vi "SSL Log Reader.vi"(9 "Slide":i64(slide) min=0 max=778291377 scale=0.0..778291377.0, 10 "Boolean 4":bool, 11 "file path (use dialog)":path=path "E:/Media/2016-07-01_cmdragons_immortals.log") -> (0 "error out":errorcluster, 1 "Playing":bool, 2 "channel 2":T1, 3 "Channel out":T1, 4 "size (in bytes)":i64, 6 "offset (in bytes)":i64)   [LabVIEW 2016]
uses:
  <extravilib>/ChannelInstances/Stream-a[.](u8)/)Channel.ctl
  <extravilib>/ChannelInstances/Stream-a[.](u8)/Write With Abort.vi
  <extravilib>/ChannelInstances/Stream-a[.](u8)/Endpoint.vi
  <extravilib>/ChannelInstances/Stream-a[.](u8)/)Channel.vi
  <resource>/ChannelSupport/_ChannelSupport/WaitIfNeeded.vi
  <extravilib>/ChannelInstances/Stream-a[.](u8).lvlib
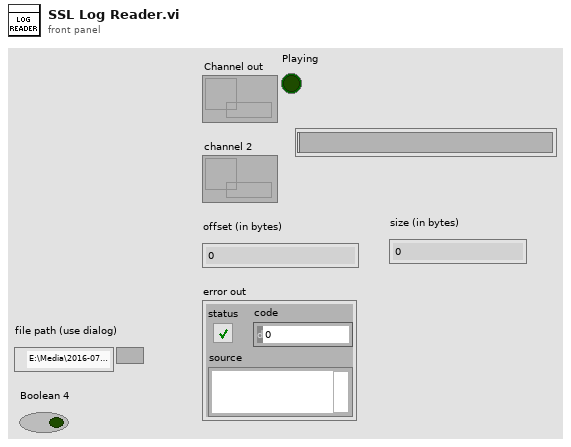
[diagram p1: front panel]
types:
  T1 = typedef "Stream-a[.](u8).lvlib/)Channel.ctl" = refnum<queue>
  T2 = enum16{"open", "replace", "create", "open or create", "replace or create", "replace or create with confirmation"}
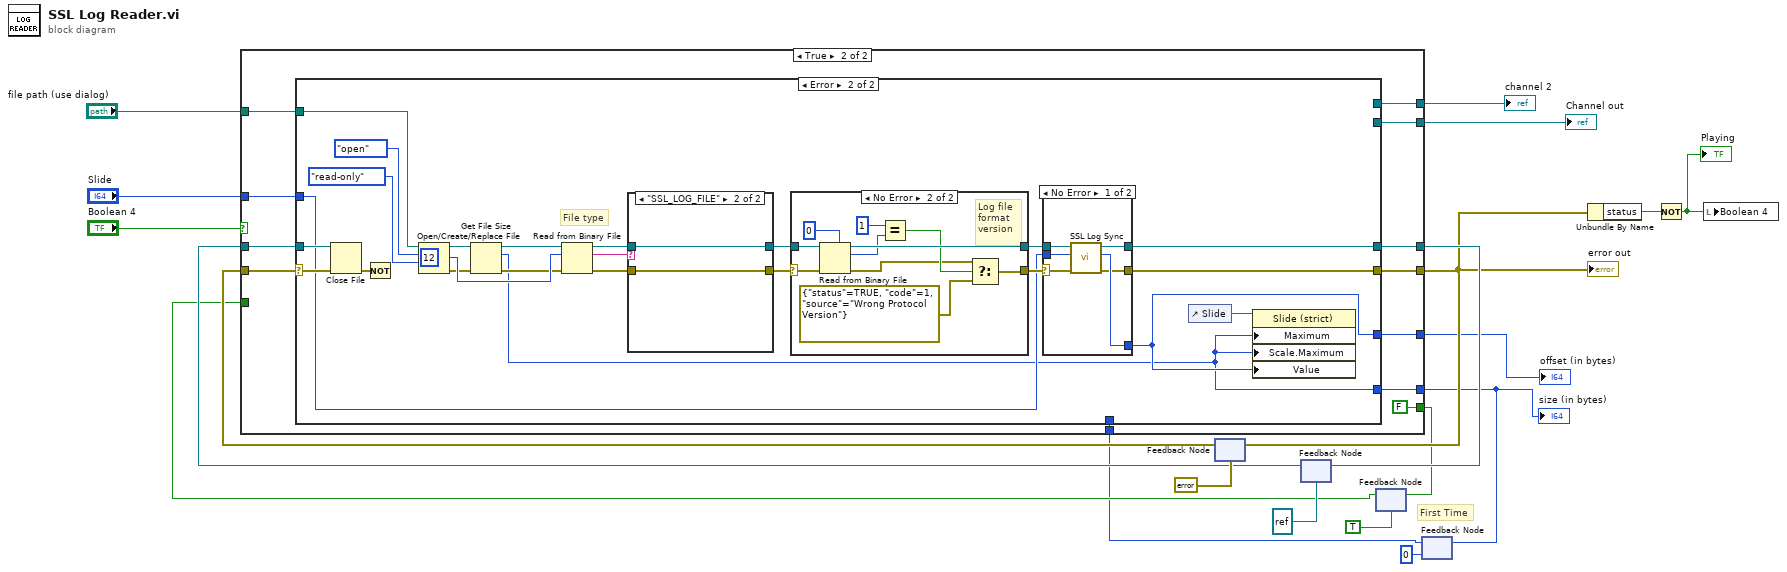
[diagram p0: block diagram]
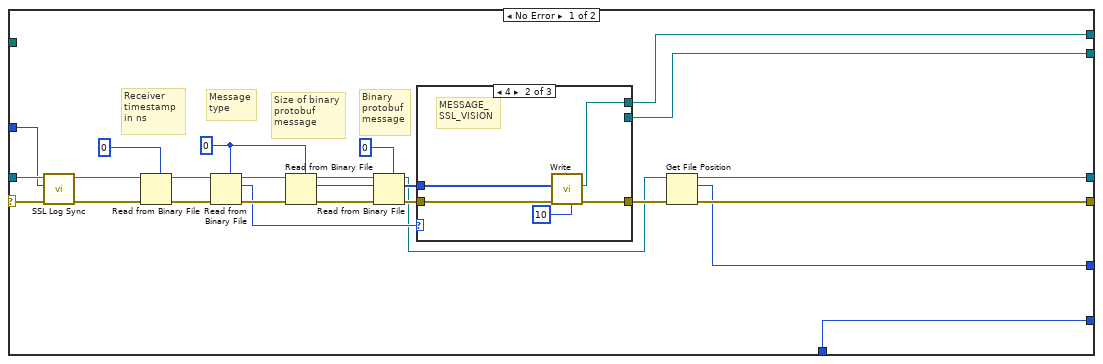
[diagram p3: hidden frame]
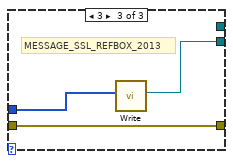
[diagram p5: hidden frame]
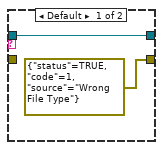
[diagram p7: hidden frame]
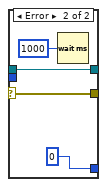
[diagram p8: hidden frame]
diagram:
  # "First Time"
  n1 = feedback #1(errorcluster {"status"=FALSE, "code"=0, "source"=""} ("error out")) -> (w13:errorcluster)
  n2 = feedback #2(refnum<file> refnum ("refnum out")) -> (w11:refnum<file>)
  n3 = feedback #3(TRUE) -> (w6:bool)
  n4 = feedback #4(i64 0 ("size (in bytes)")) -> (w1:i64)
  n5 = case shown="True" "Boolean 4" {
    tunnel: [w23 w37] -> w4
    tunnel: "file path (use dialog)" -> [_ w36]
    tunnel: [_ w35] -> w19
    tunnel: [_ w34] -> w18
    tunnel: "Slide" -> [w23 w31]
    tunnel: [w24 w33] -> w9
    tunnel: w13 -> [w24 w29]
    tunnel: [w25 w32] -> w12
    tunnel: w11 -> [w25 w30]
    tunnel: [w22 FALSE] -> w7
    tunnel: w6 -> [w22 _]
    tunnel: [w21 w27] -> w3
    tunnel: w1 -> [w21 w26]
    frame False {
    }
    frame True {
      n6 = case shown="Error" w29 {
        selector: w29 -> [w48 w78]
        tunnel: [w44 w81] -> w33
        tunnel: [w63 _] -> w34
        tunnel: [w62 _] -> w35
        tunnel: w36 -> [_ w88]
        tunnel: [w39 w74] -> w37
        tunnel: [w42 w79] -> w32
        tunnel: w30 -> [w47 w77]
        tunnel: w31 -> [w46 w75]
        tunnel: [w38 w72] -> w27
        tunnel: w26 -> [w38 _]
        frame No Error {
          w53 = 0 ("data type")
          # "Binary\nprotobuf\nmessage"
          # "Size of binary\nprotobuf \nmessage"
          # "Receiver \ntimestamp \nin ns"
          # "Message\ntype"
          n7 = call "SSL Log Sync.vi"("error in (no error)"=w48, "Slide"=w46, "Byte Stream File in"=w47) -> ("error out"=w40:errorcluster, "Byte Stream File out"=w41:refnum<file>)  [unwired: 6 in, 1 out]
          n8 = Read from Binary File(5:i64 0 ("data type"), 8:w40, 11:w41) -> (0:w58:errorcluster, 3:w59:refnum<file>)  [unwired: 3 in, 2 out]
          n9 = Read from Binary File(5:w53, 8:w58, 11:w59) -> (0:w55:errorcluster, 2:w49:i32, 3:w57:refnum<file>)  [unwired: 3 in, 1 out]
          n10 = Read from Binary File(5:w53, 8:w55, 11:w57) -> (0:w54:errorcluster, 2:w50:i32, 3:w56:refnum<file>)  [unwired: 3 in, 1 out]
          n11 = Read from Binary File(5:u8 0 ("data type"), 8:w54, 10:w50, 11:w56) -> (0:w51:errorcluster, 2:w52:u8[], 3:w43:refnum<file>)  [unwired: 2 in, 1 out]
          n12 = case shown="4" w49 {
            tunnel: w52 -> [_ w68 w70]
            tunnel: w51 -> [w64 w67 w71]
            tunnel: [w64 w67 w71] -> w45
            tunnel: [_ w66 _] -> w63
            tunnel: [_ _ w69] -> w62
            frame Default {
            }
            frame 4 {
              # "MESSAGE_\nSSL_VISION"
              n13 = call <extravilib>:"Write.vi"("size (unlimited)"=10, "element"=w68) -> ("channel"=w66:T1)  [unwired: 7 in, 2 out]
            }
            frame 3 {
              # "MESSAGE_SSL_REFBOX_2013"
              n14 = call <extravilib>:"Write.vi"("element"=w70) -> ("channel"=w69:T1)  [unwired: 8 in, 2 out]
            }
          }
          n15 = Get File Position(4:w45, 7:w43) -> (0:w44:errorcluster, 2:w39:i64, 3:w42:refnum<file>)
        }
        frame Error {
          # "File type"
          n16 = Close File(refnum=w77, error in=w78) -> (error out=w76:errorcluster)  [unwired: 1 out]
          n17 = Not(x=w76) -> ()  [unwired: 1 out]
          n18 = Open/Create/Replace File(file path (use dialog)=w88, operation (0:open)=T2."open", access (0:read/write)=enum16{"read/write", "read-only", "write-only"}."read-only") -> (refnum out=w92:refnum<file>, error out=w89:errorcluster)  [unwired: 3 in, 1 out]
          n19 = Get File Size(file=w92, error in=w89) -> (refnum out=w91:refnum<file>, size (in bytes)=w72:i64, 0:w90:errorcluster)
          n20 = Read from Binary File(8:w90, 10:12 ("count (1)"), 11:w91) -> (0:w86:errorcluster, 2:w87:string, 3:w83:refnum<file>)  [unwired: 3 in, 1 out]
          n21 = case shown="\"SSL_LOG_FILE\"" w87 {
            tunnel: w86 -> [_ w111]
            tunnel: [errorcluster {"status"=TRUE, "code"=1, "source"="Wrong File Type"} ("error out") w111] -> w85
            tunnel: [w108 w110] -> w84
            tunnel: w83 -> [w108 w110]
            frame Default {
            }
            frame "SSL_LOG_FILE" {
            }
          }
          n22 = case shown="No Error" w85 {
            selector: w85 -> [w97 w106]
            tunnel: [w97 w101] -> w82
            tunnel: w84 -> [w96 w105]
            tunnel: [w96 w104] -> w80
            frame Error {
            }
            frame No Error {
              # "Log file \nformat \nversion"
              n23 = Read from Binary File(5:0 ("prompt (Open existing file)"), 8:w106, 11:w105) -> (0:w99:errorcluster, 2:w103:i32, 3:w104:refnum<file>)  [unwired: 3 in, 1 out]
              n24 = Equal?(x=1, y=w103) -> (x = y?=w100:bool)
              n25 = Select(t=w99, s=w100, f=errorcluster {"status"=TRUE, "code"=1, "source"="Wrong Protocol Version"} ("error out")) -> (s? t:f=w101:errorcluster)
            }
          }
          n26 = case shown="No Error" w82 {
            selector: w82 -> [w117 w121]
            tunnel: [w113 w121] -> w81
            tunnel: w80 -> [w116 w120]
            tunnel: [w115 w120] -> w79
            tunnel: [w114 i64 0 ("offset (in bytes)")] -> w74
            tunnel: w75 -> [w112 _]
            frame No Error {
              n27 = call "SSL Log Sync.vi"("error in (no error)"=w117, "Slide"=w112, "Byte Stream File in"=w116) -> ("error out"=w113:errorcluster, "Offset"=w114:i64, "Byte Stream File out"=w115:refnum<file>)  [unwired: 6 in]
            }
            frame Error {
              n28 = Wait (ms)(milliseconds to wait=u32 1000) -> ()  [unwired: 1 out]
            }
          }
          n29 = control-ref of="Slide"() -> (w73:refnum<vi>)
          n30 = property on="Property Node" class="Slide (strict)"(reference=w73, "Maximum"=w72, "Scale.Maximum"=w72, "Value"=w74) -> ()  [unwired: 1 in, 2 out]
        }
      }
    }
  }
  "offset (in bytes)" <- w4
  "Channel out" <- w19
  "channel 2" <- w18
  "error out" <- w9
  "size (in bytes)" <- w3
  n31 = feedback-in #1(w9) -> ()
  n32 = feedback-in #2(w12) -> ()
  n33 = feedback-in #3(w7) -> ()
  n34 = feedback-in #4(w3) -> ()
  n35 = Unbundle By Name(w9) -> ("status"=w15:bool)
  n36 = Not(x=w15) -> (.not. x?=w16:bool)
  "Playing" <- w16
  n37 = local write "Boolean 4"(w16) -> ()
